vi "EIP Read Tags.vi"(6 "Tag Data":T4[](array[typedef]) {"Device Reference" format="%.0x"}, 7 "Device Settings":T2, 8 "error in":errorcluster, 9 "Session In":T1, 10 "Device Outputs In":dbl[](array[numeric]), 11 "Device Outputs FIFO":refnum<k33>) -> (0 "error out":errorcluster, 1 "Session Out":T1, 2 "Device Outputs Out":dbl[](array[numeric]))   [LabVIEW 2023, in "Ethernet IP Custom Device Custom Device.lvlib"]
uses:
  Ethernet IP Custom Device Custom Device.lvlib
  EIP Tag Information.ctl
  <vilib>/NI VeriStand/Custom Device API/Custom Device Item Info.ctl
  <vilib>/NI VeriStand/Custom Device API/Custom Device Item Ref.ctl
  L5K Data Types.ctl
  EIP Attribute Channel Info.ctl
  EIP Attribute Direction.ctl
  EIP Device Settings.ctl
  EIP Message Type.ctl
  <vilib>/ethernetip/ethernetip.llb/ethernetip.ctl
  <vilib>/ethernetip/ethernetip.llb/EthernetIP Tag Read INT.vi
  <vilib>/ethernetip/ethernetip.llb/EthernetIP Tag Read DINT.vi
  <vilib>/ethernetip/ethernetip.llb/EthernetIP Tag Read REAL.vi
  <vilib>/ethernetip/ethernetip.llb/EthernetIP Tag Read BOOL.vi
  <vilib>/ethernetip/ethernetip.llb/EthernetIP Tag Read SINT.vi
  <vilib>/ethernetip/ethernetip.lvlib
  <vilib>/NI VeriStand/Custom Device API/Custom Device API.lvlib
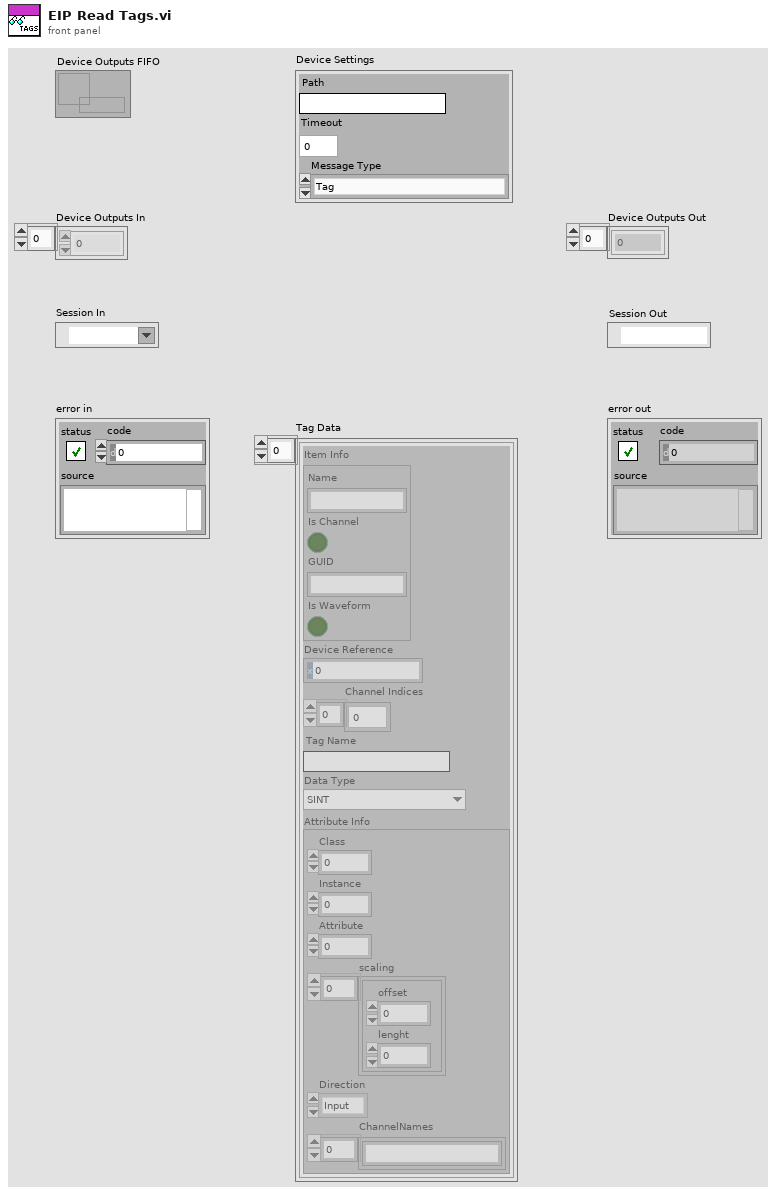
[diagram p1: front panel]
types:
  T1 = typedef "ethernetip.lvlib/ethernetip.ctl" = refnum<k21>
  T2 = typedef "Ethernet IP Custom Device Custom Device.lvlib/EIP Device Settings.ctl" = cluster{"Path":string, "Timeout":i32, "Message Type":T3}
  T3 = typedef "Ethernet IP Custom Device Custom Device.lvlib/EIP Message Type.ctl" = enum16{"Tag", "Assembly"}
  T4 = typedef "Ethernet IP Custom Device Custom Device.lvlib/EIP Tag Information.ctl" = cluster{"Item Info":T5, "Device Reference":T6, "Channel Indices":i32[], "Tag Name":string, "Data Type":T7, "Attribute Info":T8}
  T5 = typedef "Custom Device API.lvlib/Custom Device Item Info.ctl" = cluster{"Name":string, "Is Channel":bool, "GUID":string, "Is Waveform":bool}
  T6 = typedef "Custom Device API.lvlib/Custom Device Item Ref.ctl" = u64
  T7 = typedef "Ethernet IP Custom Device Custom Device.lvlib/L5K Data Types.ctl" = enum16{"SINT", "INT", "DINT", "REAL", "BOOL"}
  T8 = typedef "Ethernet IP Custom Device Custom Device.lvlib/EIP Attribute Channel Info.ctl" = cluster{"Class":i32, "Instance":u32, "Attribute":i32, "scaling":cluster{"offset":u32, "lenght":u32}[], "Direction":T9, "ChannelNames":string[]}
  T9 = typedef "Ethernet IP Custom Device Custom Device.lvlib/EIP Attribute Direction.ctl" = enum16{"Input", "Output"}
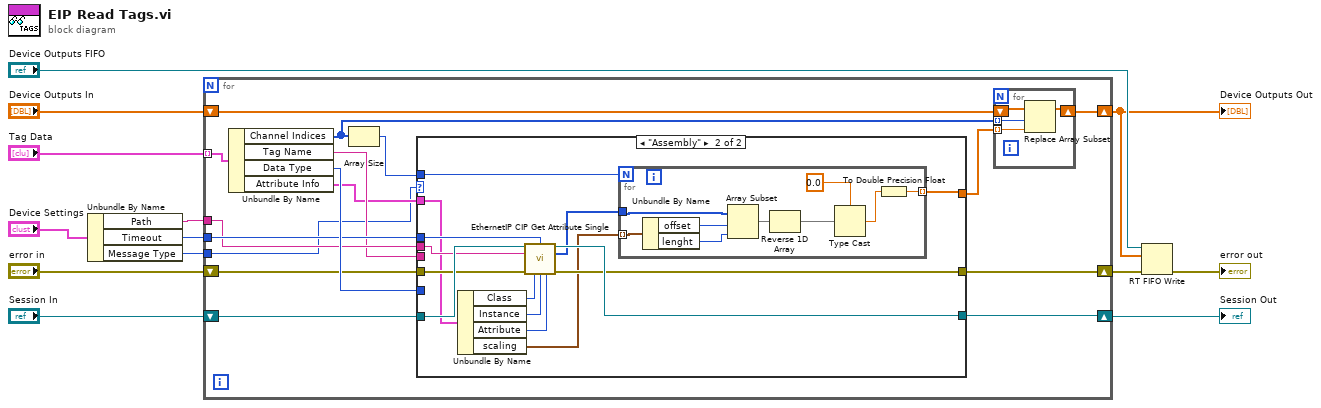
[diagram p0: block diagram]
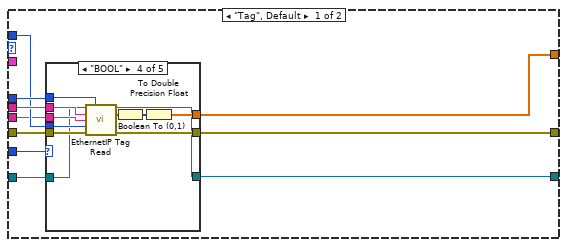
[diagram p2: hidden frame]
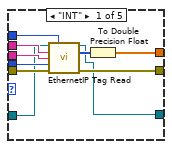
[diagram p3: hidden frame]
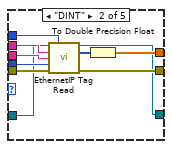
[diagram p4: hidden frame]
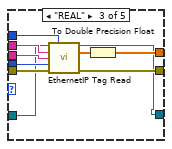
[diagram p5: hidden frame]
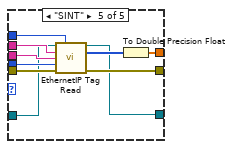
[diagram p6: hidden frame]
diagram:
  n1 = Unbundle By Name("Device Settings") -> ("Path"=w9:string, "Timeout"=w8:i32, "Message Type"=w1:T3)
  n2 = for {
    shift-right: [w20] -> w4
    shift-left: "Device Outputs In" -> [w21]
    tunnel: "Tag Data" -> [w29] mode=indexing
    shift-right: [w26] -> w6
    shift-left: "error in" -> [w27]
    tunnel: w9 -> [w24]
    tunnel: w8 -> [w25]
    shift-right: [w16] -> w2
    shift-left: "Session In" -> [w17]
    tunnel: w1 -> [w14]
    n3 = Unbundle By Name(w29) -> ("Channel Indices"=w19:i32[], "Tag Name"=w22:string, "Data Type"=w28:T7, "Attribute Info"=w15:T8)
    n4 = Array Size(array=w19) -> (size(s)=w23:i32)
    n5 = case shown="\"Assembly\"" w14 {
      tunnel: w28 -> [w39 _]
      tunnel: w27 -> [w38 w102]
      tunnel: [w37 w101] -> w26
      tunnel: w25 -> [w36 w100]
      tunnel: w24 -> [w35 w99]
      tunnel: w23 -> [w34 w94]
      tunnel: w22 -> [w33 _]
      tunnel: [w32 w91] -> w18
      tunnel: w17 -> [w31 w104]
      tunnel: [w30 w103] -> w16
      tunnel: w15 -> [_ w98]
      frame "Tag", Default {
        n6 = case shown="\"BOOL\"" w39 {
          tunnel: w34 -> [w45 w55 w65 w77 w87]
          tunnel: [w48 w58 w68 w79 w82] -> w37
          tunnel: [w47 w57 w67 w72 w89] -> w32
          tunnel: w35 -> [w46 w56 w66 w78 w88]
          tunnel: w33 -> [w44 w54 w64 w76 w84]
          tunnel: w38 -> [w43 w53 w63 w75 w86]
          tunnel: w36 -> [w42 w52 w62 w74 w85]
          tunnel: w31 -> [w40 w51 w61 w70 w83]
          tunnel: [w41 w50 w60 w71 w81] -> w30
          frame "INT" {
            n7 = call-poly <vilib>:"EthernetIP Tag Read.vi"("Session in"=w40, "Timeout (ms)"=w42, "Network Path"=w46, "Tag Name"=w44, "Number of Elements"=w45, "error in"=w43) -> ("Session out"=w41:T1, "Data"=w49:i16[], "error out"=w48:errorcluster)  [unwired: 7 in]
            n8 = To Double Precision Float(number=w49) -> (double precision float=w47:dbl[])
          }
          frame "DINT" {
            n9 = call-poly <vilib>:"EthernetIP Tag Read.vi"("Session in"=w51, "Timeout (ms)"=w52, "Network Path"=w56, "Tag Name"=w54, "Number of Elements"=w55, "error in"=w53) -> ("Session out"=w50:T1, "Data"=w59:i32[], "error out"=w58:errorcluster)  [unwired: 7 in]
            n10 = To Double Precision Float(number=w59) -> (double precision float=w57:dbl[])
          }
          frame "REAL" {
            n11 = call-poly <vilib>:"EthernetIP Tag Read.vi"("Session in"=w61, "Timeout (ms)"=w62, "Network Path"=w66, "Tag Name"=w64, "Number of Elements"=w65, "error in"=w63) -> ("Session out"=w60:T1, "Data"=w69:sgl[], "error out"=w68:errorcluster)  [unwired: 7 in]
            n12 = To Double Precision Float(number=w69) -> (double precision float=w67:dbl[])
          }
          frame "BOOL" {
            n13 = call-poly <vilib>:"EthernetIP Tag Read.vi"("Session in"=w70, "Timeout (ms)"=w74, "Network Path"=w78, "Tag Name"=w76, "Number of Elements"=w77, "error in"=w75) -> ("Session out"=w71:T1, "Data"=w80:bool[], "error out"=w79:errorcluster)  [unwired: 7 in]
            n14 = Boolean To (0,1)(Boolean=w80) -> (0, 1=w73:i16[])
            n15 = To Double Precision Float(number=w73) -> (double precision float=w72:dbl[])
          }
          frame "SINT" {
            n16 = call-poly <vilib>:"EthernetIP Tag Read.vi"("Session in"=w83, "Timeout (ms)"=w85, "Network Path"=w88, "Tag Name"=w84, "Number of Elements"=w87, "error in"=w86) -> ("Session out"=w81:T1, "Data"=w90:i8[], "error out"=w82:errorcluster)  [unwired: 7 in]
            n17 = To Double Precision Float(number=w90) -> (double precision float=w89:dbl[])
          }
        }
      }
      frame "Assembly" {
        n18 = Unbundle By Name(w98) -> ("Class"=w97:i32, "Instance"=w96:u32, "Attribute"=w95:i32, "scaling"=w93:cluster{"offset":u32, "lenght":u32}[])
        n19 = call <vilib>:"EthernetIP CIP Get Attribute Single.vi"("Session in"=w104, "Timeout (ms)"=w100, "Network Path"=w99, "error in"=w102, "Class"=w97, "Instance"=w96, "Attribute"=w95) -> ("Session out"=w103:T1, "Data"=w92:u8[], "error out"=w101:errorcluster)  [unwired: 6 in]
        n20 = for {
          N: w94 -> [_]
          tunnel: w93 -> [w112] mode=indexing
          tunnel: w92 -> [w108]
          tunnel: [w113] -> w91 mode=indexing
          n21 = Unbundle By Name(w112) -> ("offset"=w107:u32, "lenght"=w106:u32)
          n22 = Array Subset(array=w108, index=w107, length=w106) -> (w110:u8[])
          n23 = Reverse 1D Array(array=w110) -> (reversed array=w111:u8[])
          n24 = Type Cast(type=sgl 0.0, x=w111) -> (*(type *) &x=w105:sgl)
          n25 = To Double Precision Float(number=w105) -> (double precision float=w113:dbl)
        }
      }
    }
    n26 = for {
      tunnel: w18 -> [w115] mode=indexing
      tunnel: w19 -> [w116] mode=indexing
      shift-right: [w114] -> w20
      shift-left: w21 -> [w117]
      n27 = Replace Array Subset(array=w117, new element=w115, index=w116) -> (w114:dbl[])
    }
  }
  "Device Outputs Out" <- w4
  "Session Out" <- w2
  n28 = RT FIFO Write(0:"Device Outputs FIFO", 1:w4, 3:w6) -> (11:→"error out":errorcluster)  [unwired: 1 in, 4 out]
